vi "Pixie4SetUserPar.vi"(5 "Channel number":u16=2 max=3 step=1, 7 "Module number":u16 max=17 step=1, 10 "DownloadUserPar":bool, 11 "UploadUserPar":bool) -> (1 "trigger":bool, 2 "gain":dbl, 3 "Coincidence Pattern":u16=2048 format="%x")   [LabVIEW 2016]
uses:
  Drivers/Pixie4DLL.dll
panel:
  in  "?":bool
  in  "Module parameters":T1(tab)
  in  "Range":dbl=1.0 min=1.0 max=6.0 step=1.0
  out "Minimum coincidence\nwindow width [ns]":dbl=13.333333333333334 min=0.0
  in  "1 1 1 1":bool=TRUE
  in  "1 1 1 0":bool
  in  "1 1 0 1":bool
  in  "1 1 0 0":bool
  in  "1 0 1 1":bool=TRUE
  in  "1 0 1 0":bool
  in  "1 0 0 1":bool
  in  "1 0 0 0":bool
  in  "0 1 1 1":bool
  in  "0 1 1 0":bool
  in  "0 1 0 1":bool
  in  "0 1 0 0":bool
  in  "0 0 1 1":bool
  in  "0 0 1 0":bool
  in  "0 0 0 1":bool
  in  "0 0 0 0":bool
  in  "Actual coincidence\nwindow width [ns]":dbl=5000.0 min=0.0
  in  "CW options":dbl min=0.0 max=2.0 step=1.0
  in  "Module's local test adds to global test (local fail causes global fail)":bool
  in  "Accept event if global hit pattern passes global test (in PDM)":bool
  in  "Accept event if local pattern passes local test":bool=TRUE
  in  "PDM control pattern":i32 min=0 max=65535 step=1 format="%x"
  in  "Send local hit pattern to PDM in slot 2":bool
  in  "Module writes control pattern to PDM to immediate left":bool
  in  "Front panel contributes to STATUS line (wire-OR)":bool
  in  "Trigger share mode":i32 min=0 max=3 step=1
  in  "Front panel drives GFLT line (one module only)":bool
  in  "32 buffers per spill":bool=TRUE
  in  "Channel parameters":T2(tab)=enum."Analog signal conditioning"
  in  "Threshold":dbl=10.0 min=0.0
  in  "Flat top [µs]":dbl=0.08 min=0.0 max=0.8533 step=0.013333
  in  "Rise time [µs]":dbl=0.76 min=0.02666 max=0.8533 step=0.0133
  in  "Flat top [µs]":dbl=0.29333333333333333 min=0.0
  in  "Rise time [µs]":dbl=3.0933333333333337 min=0.0266 max=105.813
  in  "Integrator":dbl min=0.0 max=5.0 step=1.0
  in  "Inverted":bool
  in  "Estimate energy if not hit":bool
  in  "Latch local timestamp even in group trigger mode":bool
  in  "Threshold [%]":dbl=25.0 min=0.0 max=100.0 step=1.0
  in  "Compute constant fraction timing":bool
  in  "Histogram energies":bool=TRUE
  in  "GFLT required":bool
  in  "Trigger positive":bool=TRUE
  in  "Enable trigger":bool=TRUE
  in  "Read always":bool=TRUE
  in  "Good channel":bool=TRUE
  in  "Allow negative energy":bool
  in  "Respond to group triggers only":bool
  in  "Invert the GATE polarity to start the GATE Window":bool
  in  "Pause pileup inspection":bool
  in  "Invert pileup inspection":bool
  in  "Ignore out-of-range":bool
  in  "Disable pileup inspection":bool
  in  "Route VETO signal to be used for GATE":bool
  in  "Invert GATE polarity for acceptance":bool
  in  "GATE signal required to accept events":bool
  in  "PSA End [µs]":dbl min=0.0
  in  "PSA Start [µs]":dbl min=0.0
  in  "Delay [µs]":dbl min=0.0
  in  "Trace length [µs]":dbl min=0.0
  in  "Offset [V]":dbl=0.1180267333984375 min=0.0
  in  "Gain [V/V]":dbl=2.0 min=0.0
  in  "Tau [µs]":dbl=50.0 min=0.0
  in  "Binning factor":dbl=1.0 min=1.0 max=6.0 step=1.0
  in  "Minimum energy":dbl min=0.0
  in  "Gate Delay [µs]":dbl=0.013333333333333334 step=0.013333
  in  "Gate Window [µs]":dbl=0.013333333333333334 step=0.013333
  in  "Baseline Averaging":dbl=65534.0 min=0.0 max=65535.0 step=1.0
  in  "Baseline Cut":dbl=58.0 min=0.0 max=65535.0 step=1.0
  # "(Must also enable Upload button)"
  # "Energy Filter"
  # "Edit required hit patterns"
  # "Channels"
  # "Channels"
  # "3 2 1 0"
  # "3 2 1 0"
  # "0x"
  # "0: Increase for energy filter, never decrease\n1: Keep at required energy filter width\n2: Disregard energy filter requirement"
  # "0x"
  # "Trigger Filter"
  # "Energy Filter"
  # "Edit Channel Control Register A"
  # "Edit Channel Control Register C"
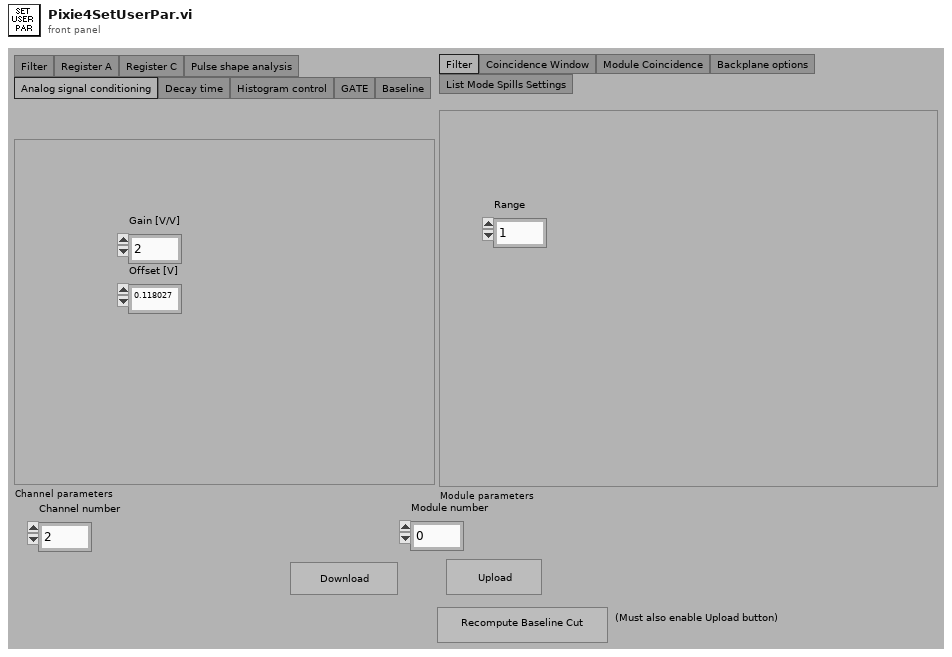
[diagram p1: front panel]
types:
  T1 = enum32{"Filter", "Coincidence Window", "Module Coincidence", "Backplane options", "List Mode Spills Settings"}
  T2 = enum32{"Filter", "Register A", "Register C", "Pulse shape analysis", "Analog signal conditioning", "Decay time", "Histogram control", "GATE", "Baseline"}
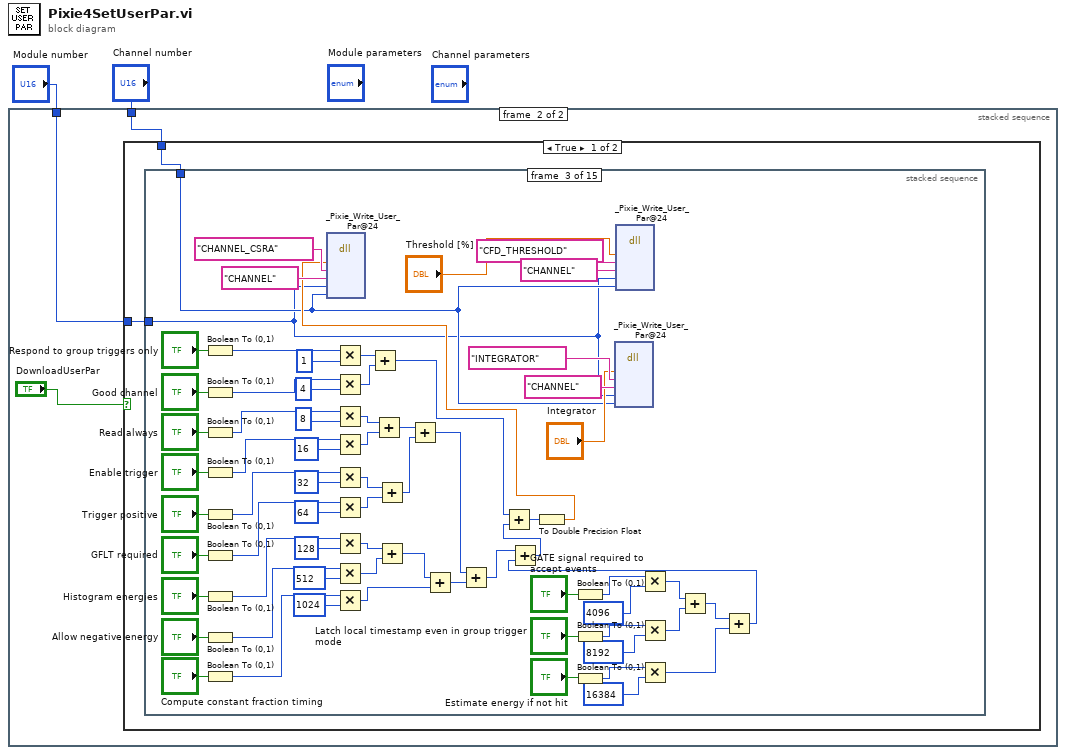
[diagram p0: block diagram]
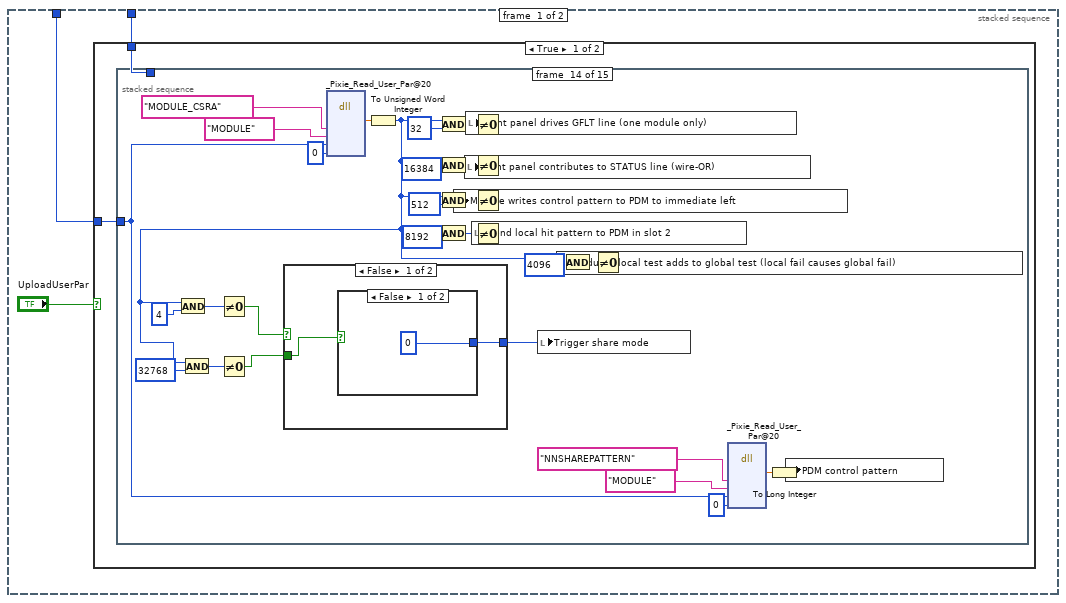
[diagram p2: hidden frame]
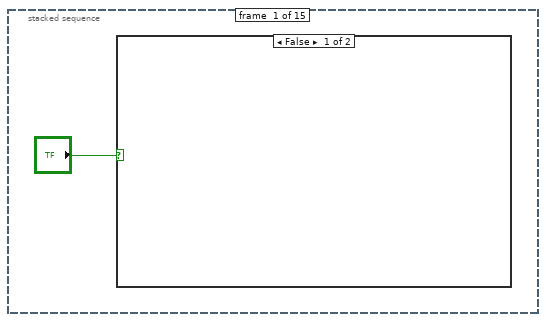
[diagram p3: hidden frame]
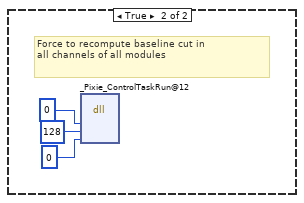
[diagram p4: hidden frame]
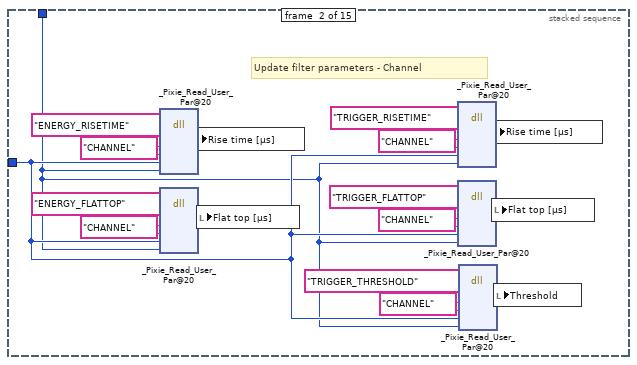
[diagram p5: hidden frame]
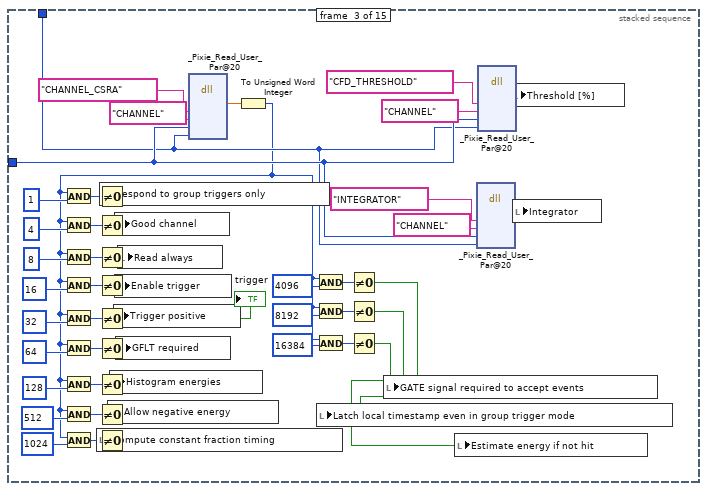
[diagram p6: hidden frame]
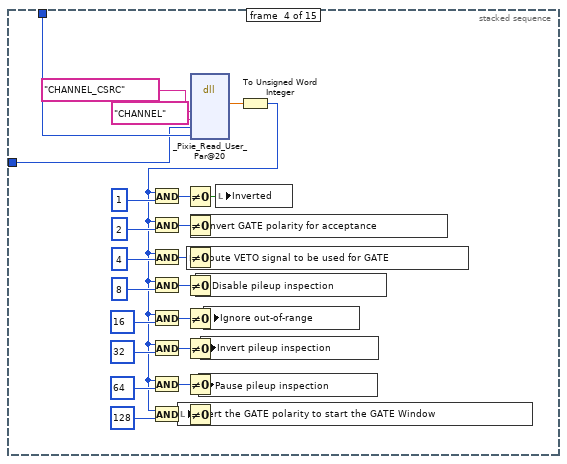
[diagram p7: hidden frame]
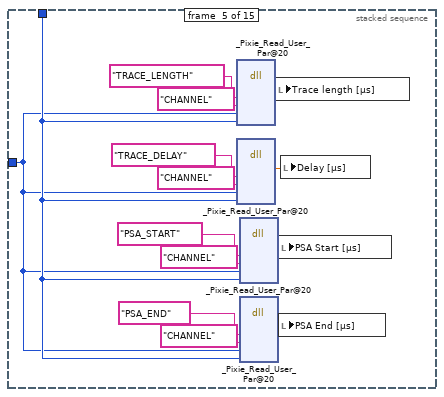
[diagram p8: hidden frame]
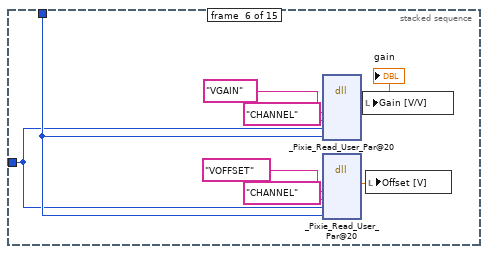
[diagram p9: hidden frame]
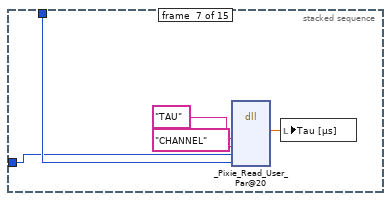
[diagram p10: hidden frame]
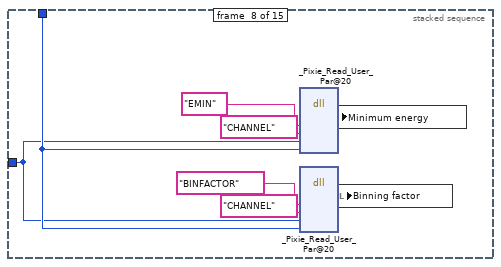
[diagram p11: hidden frame]
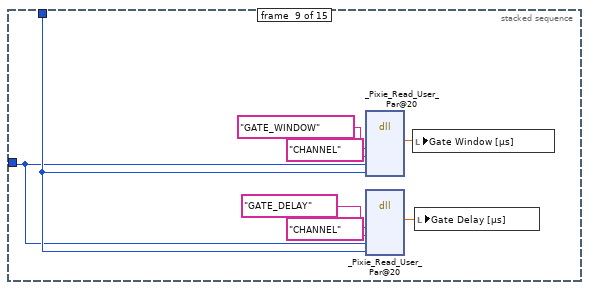
[diagram p12: hidden frame]
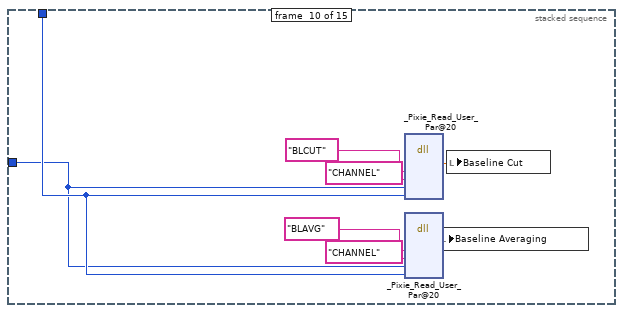
[diagram p13: hidden frame]
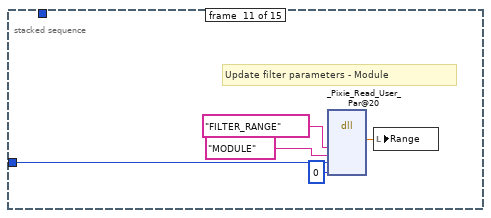
[diagram p14: hidden frame]
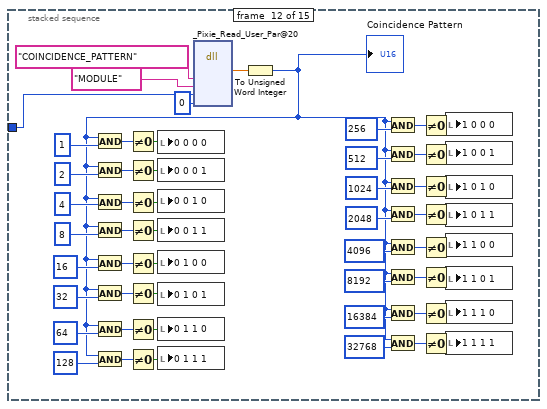
[diagram p15: hidden frame]
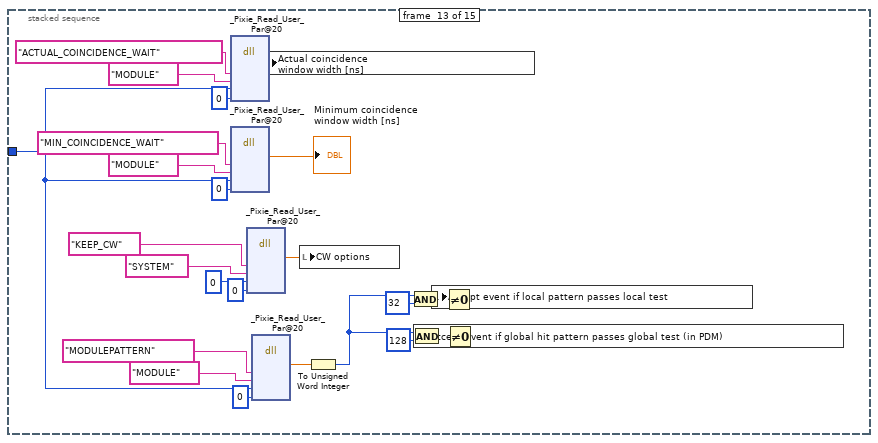
[diagram p16: hidden frame]
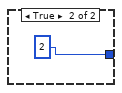
[diagram p17: hidden frame]
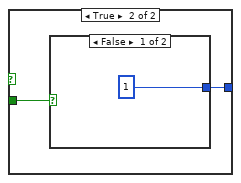
[diagram p18: hidden frame]
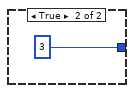
[diagram p19: hidden frame]
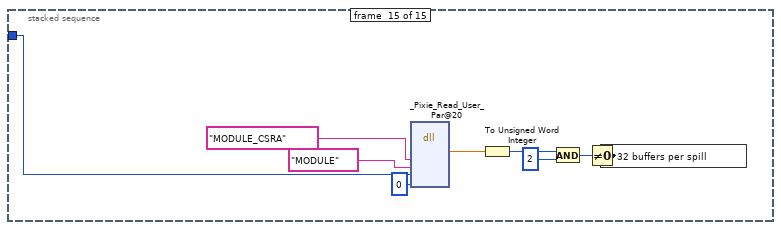
[diagram p20: hidden frame]
diagram:
  n1 = stacked-sequence {
    tunnel: "Module number" -> [w4 w294]
    tunnel: "Channel number" -> [w3 w293]
    frame #0 {
      n2 = case shown="True" "UploadUserPar" {
        tunnel: w4 -> [w7 _]
        tunnel: w3 -> [w6 _]
        frame True {
          n3 = stacked-sequence {
            tunnel: w7 -> [_ w14 w48 w86 w111 w123 w130 w136 w144 w156 w160 w213 w228 w254 w288]
            tunnel: w6 -> [_ w13 w47 w87 w112 w124 w131 w137 w145 w157 _ _ _ _ _]
            frame #0 {
              n4 = case shown="False" "?" {
                frame False {
                }
                frame True {
                  # "Force to recompute baseline cut in\nall channels of all modules"
                  n5 = dll-call lib="D:/Users/wymanm/Desktop/DAQuiri - 2017a/lois/Drivers/Pixie4DLL.dll" fn="_Pixie_ControlTaskRun@12"("ModNum"=0, "ControlTask"=128, "MaxPoll"=0) -> ()  [unwired: 7 in, 2 out]
                }
              }
            }
            frame #1 {
              # "Update filter parameters - Channel"
              n6 = dll-call lib="D:/Users/wymanm/Desktop/DAQuiri - 2017a/lois/Drivers/Pixie4DLL.dll" fn="_Pixie_Read_User_Par@20"("User_Par_Name"="ENERGY_RISETIME", "User_Par_Type"="CHANNEL", "ModNum"=w14, "ChanNum"=w13) -> ("User_Par_Value"=w26:dbl)  [unwired: 9 in, 2 out]
              n7 = dll-call lib="D:/Users/wymanm/Desktop/DAQuiri - 2017a/lois/Drivers/Pixie4DLL.dll" fn="_Pixie_Read_User_Par@20"("User_Par_Name"="ENERGY_FLATTOP", "User_Par_Type"="CHANNEL", "ModNum"=w14, "ChanNum"=w13) -> ("User_Par_Value"=w23:dbl)  [unwired: 9 in, 2 out]
              n8 = local write "Rise time [µs]"(w26) -> ()
              n9 = local write "Flat top [µs]"(w23) -> ()
              n10 = dll-call lib="D:/Users/wymanm/Desktop/DAQuiri - 2017a/lois/Drivers/Pixie4DLL.dll" fn="_Pixie_Read_User_Par@20"("User_Par_Name"="TRIGGER_RISETIME", "User_Par_Type"="CHANNEL", "ModNum"=w14, "ChanNum"=w13) -> ("User_Par_Value"=w18:dbl)  [unwired: 9 in, 2 out]
              n11 = dll-call lib="D:/Users/wymanm/Desktop/DAQuiri - 2017a/lois/Drivers/Pixie4DLL.dll" fn="_Pixie_Read_User_Par@20"("User_Par_Name"="TRIGGER_FLATTOP", "User_Par_Type"="CHANNEL", "ModNum"=w14, "ChanNum"=w13) -> ("User_Par_Value"=w17:dbl)  [unwired: 9 in, 2 out]
              n12 = dll-call lib="D:/Users/wymanm/Desktop/DAQuiri - 2017a/lois/Drivers/Pixie4DLL.dll" fn="_Pixie_Read_User_Par@20"("User_Par_Name"="TRIGGER_THRESHOLD", "User_Par_Type"="CHANNEL", "ModNum"=w14, "ChanNum"=w13) -> ("User_Par_Value"=w12:dbl)  [unwired: 9 in, 2 out]
              n13 = local write "Rise time [µs]"(w18) -> ()
              n14 = local write "Flat top [µs]"(w17) -> ()
              n15 = local write "Threshold"(w12) -> ()
            }
            frame #2 {
              n16 = dll-call lib="D:/Users/wymanm/Desktop/DAQuiri - 2017a/lois/Drivers/Pixie4DLL.dll" fn="_Pixie_Read_User_Par@20"("User_Par_Name"="CHANNEL_CSRA", "User_Par_Type"="CHANNEL", "ModNum"=w48, "ChanNum"=w47) -> ("User_Par_Value"=w68:dbl)  [unwired: 9 in, 2 out]
              n17 = To Unsigned Word Integer(number=w68) -> (unsigned 16bit integer=w32:u16)
              n18 = And(x=w32, y=1) -> (x .and. y?=w66:i32)
              n19 = And(x=w32, y=4) -> (x .and. y?=w63:i32)
              n20 = And(x=w32, y=8) -> (x .and. y?=w61:i32)
              n21 = And(x=w32, y=16) -> (x .and. y?=w59:i32)
              n22 = And(x=w32, y=32) -> (x .and. y?=w57:i32)
              n23 = And(x=w32, y=64) -> (x .and. y?=w55:i32)
              n24 = And(x=w32, y=128) -> (x .and. y?=w53:i32)
              n25 = And(x=w32, y=512) -> (x .and. y?=w51:i32)
              n26 = And(x=w32, y=1024) -> (x .and. y?=w49:i32)
              n27 = Not Equal To 0?(x=w66) -> (x != 0?=w65:bool)
              n28 = Not Equal To 0?(x=w63) -> (x != 0?=w46:bool)
              n29 = Not Equal To 0?(x=w61) -> (x != 0?=w45:bool)
              n30 = Not Equal To 0?(x=w59) -> (x != 0?=w44:bool)
              n31 = Not Equal To 0?(x=w57) -> (x != 0?=w43:bool)
              "trigger" <- w43
              n32 = Not Equal To 0?(x=w55) -> (x != 0?=w42:bool)
              n33 = Not Equal To 0?(x=w53) -> (x != 0?=w41:bool)
              n34 = Not Equal To 0?(x=w51) -> (x != 0?=w40:bool)
              n35 = Not Equal To 0?(x=w49) -> (x != 0?=w39:bool)
              n36 = local write "Compute constant fraction timing"(w39) -> ()
              n37 = local write "Respond to group triggers only"(w65) -> ()
              n38 = local write "Allow negative energy"(w40) -> ()
              n39 = local write "Histogram energies"(w41) -> ()
              n40 = local write "Trigger positive"(w43) -> ()
              n41 = local write "Good channel"(w46) -> ()
              n42 = local write "Enable trigger"(w44) -> ()
              n43 = local write "GFLT required"(w42) -> ()
              n44 = local write "Read always"(w45) -> ()
              n45 = And(x=w32, y=4096) -> (x .and. y?=w37:i32)
              n46 = And(x=w32, y=8192) -> (x .and. y?=w35:i32)
              n47 = And(x=w32, y=16384) -> (x .and. y?=w33:i32)
              n48 = Not Equal To 0?(x=w37) -> (x != 0?=w31:bool)
              n49 = Not Equal To 0?(x=w35) -> (x != 0?=w30:bool)
              n50 = local write "Latch local timestamp even in group trigger mode"(w30) -> ()
              n51 = Not Equal To 0?(x=w33) -> (x != 0?=w29:bool)
              n52 = local write "GATE signal required to accept events"(w31) -> ()
              n53 = local write "Estimate energy if not hit"(w29) -> ()
              n54 = dll-call lib="D:/Users/wymanm/Desktop/DAQuiri - 2017a/lois/Drivers/Pixie4DLL.dll" fn="_Pixie_Read_User_Par@20"("User_Par_Name"="INTEGRATOR", "User_Par_Type"="CHANNEL", "ModNum"=w48, "ChanNum"=w47) -> ("User_Par_Value"=w69:dbl)  [unwired: 9 in, 2 out]
              n55 = dll-call lib="D:/Users/wymanm/Desktop/DAQuiri - 2017a/lois/Drivers/Pixie4DLL.dll" fn="_Pixie_Read_User_Par@20"("User_Par_Name"="CFD_THRESHOLD", "User_Par_Type"="CHANNEL", "ModNum"=w48, "ChanNum"=w47) -> ("User_Par_Value"=w70:dbl)  [unwired: 9 in, 2 out]
              n56 = local write "Threshold [%]"(w70) -> ()
              n57 = local write "Integrator"(w69) -> ()
            }
            frame #3 {
              n58 = dll-call lib="D:/Users/wymanm/Desktop/DAQuiri - 2017a/lois/Drivers/Pixie4DLL.dll" fn="_Pixie_Read_User_Par@20"("User_Par_Name"="CHANNEL_CSRC", "User_Par_Type"="CHANNEL", "ModNum"=w86, "ChanNum"=w87) -> ("User_Par_Value"=w88:dbl)  [unwired: 9 in, 2 out]
              n59 = To Unsigned Word Integer(number=w88) -> (unsigned 16bit integer=w85:u16)
              n60 = And(x=w85, y=1) -> (x .and. y?=w105:i32)
              n61 = And(x=w85, y=2) -> (x .and. y?=w103:i32)
              n62 = And(x=w85, y=4) -> (x .and. y?=w101:i32)
              n63 = And(x=w85, y=8) -> (x .and. y?=w99:i32)
              n64 = And(x=w85, y=16) -> (x .and. y?=w97:i32)
              n65 = And(x=w85, y=32) -> (x .and. y?=w95:i32)
              n66 = And(x=w85, y=64) -> (x .and. y?=w93:i32)
              n67 = And(x=w85, y=128) -> (x .and. y?=w91:i32)
              n68 = Not Equal To 0?(x=w105) -> (x != 0?=w84:bool)
              n69 = Not Equal To 0?(x=w103) -> (x != 0?=w83:bool)
              n70 = Not Equal To 0?(x=w101) -> (x != 0?=w82:bool)
              n71 = Not Equal To 0?(x=w99) -> (x != 0?=w81:bool)
              n72 = Not Equal To 0?(x=w97) -> (x != 0?=w80:bool)
              n73 = Not Equal To 0?(x=w95) -> (x != 0?=w79:bool)
              n74 = Not Equal To 0?(x=w93) -> (x != 0?=w78:bool)
              n75 = Not Equal To 0?(x=w91) -> (x != 0?=w77:bool)
              n76 = local write "Invert the GATE polarity to start the GATE Window"(w77) -> ()
              n77 = local write "Route VETO signal to be used for GATE"(w82) -> ()
              n78 = local write "Invert GATE polarity for acceptance"(w83) -> ()
              n79 = local write "Disable pileup inspection"(w81) -> ()
              n80 = local write "Pause pileup inspection"(w78) -> ()
              n81 = local write "Invert pileup inspection"(w79) -> ()
              n82 = local write "Ignore out-of-range"(w80) -> ()
              n83 = local write "Inverted"(w84) -> ()
            }
            frame #4 {
              n84 = dll-call lib="D:/Users/wymanm/Desktop/DAQuiri - 2017a/lois/Drivers/Pixie4DLL.dll" fn="_Pixie_Read_User_Par@20"("User_Par_Name"="TRACE_LENGTH", "User_Par_Type"="CHANNEL", "ModNum"=w111, "ChanNum"=w112) -> ("User_Par_Value"=w110:dbl)  [unwired: 9 in, 2 out]
              n85 = dll-call lib="D:/Users/wymanm/Desktop/DAQuiri - 2017a/lois/Drivers/Pixie4DLL.dll" fn="_Pixie_Read_User_Par@20"("User_Par_Name"="TRACE_DELAY", "User_Par_Type"="CHANNEL", "ModNum"=w111, "ChanNum"=w112) -> ("User_Par_Value"=w109:dbl)  [unwired: 9 in, 2 out]
              n86 = dll-call lib="D:/Users/wymanm/Desktop/DAQuiri - 2017a/lois/Drivers/Pixie4DLL.dll" fn="_Pixie_Read_User_Par@20"("User_Par_Name"="PSA_START", "User_Par_Type"="CHANNEL", "ModNum"=w111, "ChanNum"=w112) -> ("User_Par_Value"=w108:dbl)  [unwired: 9 in, 2 out]
              n87 = dll-call lib="D:/Users/wymanm/Desktop/DAQuiri - 2017a/lois/Drivers/Pixie4DLL.dll" fn="_Pixie_Read_User_Par@20"("User_Par_Name"="PSA_END", "User_Par_Type"="CHANNEL", "ModNum"=w111, "ChanNum"=w112) -> ("User_Par_Value"=w107:dbl)  [unwired: 9 in, 2 out]
              n88 = local write "Trace length [µs]"(w110) -> ()
              n89 = local write "PSA Start [µs]"(w108) -> ()
              n90 = local write "PSA End [µs]"(w107) -> ()
              n91 = local write "Delay [µs]"(w109) -> ()
            }
            frame #5 {
              n92 = dll-call lib="D:/Users/wymanm/Desktop/DAQuiri - 2017a/lois/Drivers/Pixie4DLL.dll" fn="_Pixie_Read_User_Par@20"("User_Par_Name"="VGAIN", "User_Par_Type"="CHANNEL", "ModNum"=w123, "ChanNum"=w124) -> ("User_Par_Value"=w122:dbl)  [unwired: 9 in, 2 out]
              "gain" <- w122
              n93 = dll-call lib="D:/Users/wymanm/Desktop/DAQuiri - 2017a/lois/Drivers/Pixie4DLL.dll" fn="_Pixie_Read_User_Par@20"("User_Par_Name"="VOFFSET", "User_Par_Type"="CHANNEL", "ModNum"=w123, "ChanNum"=w124) -> ("User_Par_Value"=w121:dbl)  [unwired: 9 in, 2 out]
              n94 = local write "Gain [V/V]"(w122) -> ()
              n95 = local write "Offset [V]"(w121) -> ()
            }
            frame #6 {
              n96 = dll-call lib="D:/Users/wymanm/Desktop/DAQuiri - 2017a/lois/Drivers/Pixie4DLL.dll" fn="_Pixie_Read_User_Par@20"("User_Par_Name"="TAU", "User_Par_Type"="CHANNEL", "ModNum"=w130, "ChanNum"=w131) -> ("User_Par_Value"=w129:dbl)  [unwired: 9 in, 2 out]
              n97 = local write "Tau [µs]"(w129) -> ()
            }
            frame #7 {
              n98 = dll-call lib="D:/Users/wymanm/Desktop/DAQuiri - 2017a/lois/Drivers/Pixie4DLL.dll" fn="_Pixie_Read_User_Par@20"("User_Par_Name"="EMIN", "User_Par_Type"="CHANNEL", "ModNum"=w136, "ChanNum"=w137) -> ("User_Par_Value"=w135:dbl)  [unwired: 9 in, 2 out]
              n99 = dll-call lib="D:/Users/wymanm/Desktop/DAQuiri - 2017a/lois/Drivers/Pixie4DLL.dll" fn="_Pixie_Read_User_Par@20"("User_Par_Name"="BINFACTOR", "User_Par_Type"="CHANNEL", "ModNum"=w136, "ChanNum"=w137) -> ("User_Par_Value"=w134:dbl)  [unwired: 9 in, 2 out]
              n100 = local write "Minimum energy"(w135) -> ()
              n101 = local write "Binning factor"(w134) -> ()
            }
            frame #8 {
              n102 = dll-call lib="D:/Users/wymanm/Desktop/DAQuiri - 2017a/lois/Drivers/Pixie4DLL.dll" fn="_Pixie_Read_User_Par@20"("User_Par_Name"="GATE_WINDOW", "User_Par_Type"="CHANNEL", "ModNum"=w144, "ChanNum"=w145) -> ("User_Par_Value"=w143:dbl)  [unwired: 9 in, 2 out]
              n103 = dll-call lib="D:/Users/wymanm/Desktop/DAQuiri - 2017a/lois/Drivers/Pixie4DLL.dll" fn="_Pixie_Read_User_Par@20"("User_Par_Name"="GATE_DELAY", "User_Par_Type"="CHANNEL", "ModNum"=w144, "ChanNum"=w145) -> ("User_Par_Value"=w142:dbl)  [unwired: 9 in, 2 out]
              n104 = local write "Gate Window [µs]"(w143) -> ()
              n105 = local write "Gate Delay [µs]"(w142) -> ()
            }
            frame #9 {
              n106 = dll-call lib="D:/Users/wymanm/Desktop/DAQuiri - 2017a/lois/Drivers/Pixie4DLL.dll" fn="_Pixie_Read_User_Par@20"("User_Par_Name"="BLCUT", "User_Par_Type"="CHANNEL", "ModNum"=w156, "ChanNum"=w157) -> ("User_Par_Value"=w151:dbl)  [unwired: 9 in, 2 out]
              n107 = dll-call lib="D:/Users/wymanm/Desktop/DAQuiri - 2017a/lois/Drivers/Pixie4DLL.dll" fn="_Pixie_Read_User_Par@20"("User_Par_Name"="BLAVG", "User_Par_Type"="CHANNEL", "ModNum"=w156, "ChanNum"=w157) -> ("User_Par_Value"=w150:dbl)  [unwired: 9 in, 2 out]
              n108 = local write "Baseline Averaging"(w150) -> ()
              n109 = local write "Baseline Cut"(w151) -> ()
            }
            frame #10 {
              # "Update filter parameters - Module"
              n110 = dll-call lib="D:/Users/wymanm/Desktop/DAQuiri - 2017a/lois/Drivers/Pixie4DLL.dll" fn="_Pixie_Read_User_Par@20"("User_Par_Name"="FILTER_RANGE", "User_Par_Type"="MODULE", "ModNum"=w160, "ChanNum"=0) -> ("User_Par_Value"=w158:dbl)  [unwired: 9 in, 2 out]
              n111 = local write "Range"(w158) -> ()
            }
            frame #11 {
              n112 = dll-call lib="D:/Users/wymanm/Desktop/DAQuiri - 2017a/lois/Drivers/Pixie4DLL.dll" fn="_Pixie_Read_User_Par@20"("User_Par_Name"="COINCIDENCE_PATTERN", "User_Par_Type"="MODULE", "ModNum"=w213, "ChanNum"=0) -> ("User_Par_Value"=w180:dbl)  [unwired: 9 in, 2 out]
              n113 = To Unsigned Word Integer(number=w180) -> (unsigned 16bit integer=w163:u16)
              "Coincidence Pattern" <- w163
              n114 = And(x=w163, y=1) -> (x .and. y?=w211:i32)
              n115 = And(x=w163, y=2) -> (x .and. y?=w209:i32)
              n116 = And(x=w163, y=4) -> (x .and. y?=w207:i32)
              n117 = And(x=w163, y=8) -> (x .and. y?=w205:i32)
              n118 = And(x=w163, y=16) -> (x .and. y?=w203:i32)
              n119 = And(x=w163, y=32) -> (x .and. y?=w201:i32)
              n120 = And(x=w163, y=64) -> (x .and. y?=w199:i32)
              n121 = And(x=w163, y=128) -> (x .and. y?=w197:i32)
              n122 = Not Equal To 0?(x=w211) -> (x != 0?=w179:bool)
              n123 = Not Equal To 0?(x=w209) -> (x != 0?=w178:bool)
              n124 = Not Equal To 0?(x=w207) -> (x != 0?=w177:bool)
              n125 = Not Equal To 0?(x=w205) -> (x != 0?=w176:bool)
              n126 = Not Equal To 0?(x=w203) -> (x != 0?=w175:bool)
              n127 = Not Equal To 0?(x=w201) -> (x != 0?=w174:bool)
              n128 = Not Equal To 0?(x=w199) -> (x != 0?=w173:bool)
              n129 = Not Equal To 0?(x=w197) -> (x != 0?=w172:bool)
              n130 = local write "0 0 0 0"(w179) -> ()
              n131 = local write "0 0 0 1"(w178) -> ()
              n132 = local write "0 0 1 0"(w177) -> ()
              n133 = local write "0 0 1 1"(w176) -> ()
              n134 = local write "0 1 0 0"(w175) -> ()
              n135 = local write "0 1 0 1"(w174) -> ()
              n136 = local write "0 1 1 0"(w173) -> ()
              n137 = local write "0 1 1 1"(w172) -> ()
              n138 = And(x=w163, y=256) -> (x .and. y?=w195:i32)
              n139 = And(x=w163, y=512) -> (x .and. y?=w193:i32)
              n140 = And(x=w163, y=1024) -> (x .and. y?=w191:i32)
              n141 = And(x=w163, y=2048) -> (x .and. y?=w189:i32)
              n142 = And(x=w163, y=4096) -> (x .and. y?=w187:i32)
              n143 = And(x=w163, y=8192) -> (x .and. y?=w185:i32)
              n144 = And(x=w163, y=16384) -> (x .and. y?=w183:i32)
              n145 = And(x=w163, y=32768) -> (x .and. y?=w181:i32)
              n146 = Not Equal To 0?(x=w195) -> (x != 0?=w171:bool)
              n147 = Not Equal To 0?(x=w193) -> (x != 0?=w170:bool)
              n148 = Not Equal To 0?(x=w191) -> (x != 0?=w169:bool)
              n149 = Not Equal To 0?(x=w189) -> (x != 0?=w168:bool)
              n150 = Not Equal To 0?(x=w187) -> (x != 0?=w167:bool)
              n151 = Not Equal To 0?(x=w185) -> (x != 0?=w166:bool)
              n152 = Not Equal To 0?(x=w183) -> (x != 0?=w165:bool)
              n153 = Not Equal To 0?(x=w181) -> (x != 0?=w164:bool)
              n154 = local write "1 0 0 0"(w171) -> ()
              n155 = local write "1 0 0 1"(w170) -> ()
              n156 = local write "1 0 1 0"(w169) -> ()
              n157 = local write "1 0 1 1"(w168) -> ()
              n158 = local write "1 1 0 0"(w167) -> ()
              n159 = local write "1 1 0 1"(w166) -> ()
              n160 = local write "1 1 1 0"(w165) -> ()
              n161 = local write "1 1 1 1"(w164) -> ()
            }
            frame #12 {
              n162 = dll-call lib="D:/Users/wymanm/Desktop/DAQuiri - 2017a/lois/Drivers/Pixie4DLL.dll" fn="_Pixie_Read_User_Par@20"("User_Par_Name"="ACTUAL_COINCIDENCE_WAIT", "User_Par_Type"="MODULE", "ModNum"=w228, "ChanNum"=0) -> ("User_Par_Value"=w218:dbl)  [unwired: 9 in, 2 out]
              n163 = dll-call lib="D:/Users/wymanm/Desktop/DAQuiri - 2017a/lois/Drivers/Pixie4DLL.dll" fn="_Pixie_Read_User_Par@20"("User_Par_Name"="MIN_COINCIDENCE_WAIT", "User_Par_Type"="MODULE", "ModNum"=w228, "ChanNum"=0) -> ("User_Par_Value"=→"Minimum coincidence\nwindow width [ns]":dbl)  [unwired: 9 in, 2 out]
              n164 = dll-call lib="D:/Users/wymanm/Desktop/DAQuiri - 2017a/lois/Drivers/Pixie4DLL.dll" fn="_Pixie_Read_User_Par@20"("User_Par_Name"="KEEP_CW", "User_Par_Type"="SYSTEM", "ModNum"=0, "ChanNum"=0) -> ("User_Par_Value"=w217:dbl)  [unwired: 9 in, 2 out]
              n165 = dll-call lib="D:/Users/wymanm/Desktop/DAQuiri - 2017a/lois/Drivers/Pixie4DLL.dll" fn="_Pixie_Read_User_Par@20"("User_Par_Name"="MODULEPATTERN", "User_Par_Type"="MODULE", "ModNum"=w228, "ChanNum"=0) -> ("User_Par_Value"=w225:dbl)  [unwired: 9 in, 2 out]
              n166 = local write "Actual coincidence\nwindow width [ns]"(w218) -> ()
              n167 = local write "CW options"(w217) -> ()
              n168 = To Unsigned Word Integer(number=w225) -> (unsigned 16bit integer=w221:u16)
              n169 = And(x=w221, y=32) -> (x .and. y?=w226:i32)
              n170 = And(x=w221, y=128) -> (x .and. y?=w223:i32)
              n171 = Not Equal To 0?(x=w226) -> (x != 0?=w219:bool)
              n172 = local write "Accept event if local pattern passes local test"(w219) -> ()
              n173 = Not Equal To 0?(x=w223) -> (x != 0?=w222:bool)
              n174 = local write "Accept event if global hit pattern passes global test (in PDM)"(w222) -> ()
            }
            frame #13 {
              n175 = dll-call lib="D:/Users/wymanm/Desktop/DAQuiri - 2017a/lois/Drivers/Pixie4DLL.dll" fn="_Pixie_Read_User_Par@20"("User_Par_Name"="MODULE_CSRA", "User_Par_Type"="MODULE", "ModNum"=w254, "ChanNum"=0) -> ("User_Par_Value"=w269:dbl)  [unwired: 9 in, 2 out]
              n176 = To Unsigned Word Integer(number=w269) -> (unsigned 16bit integer=w243:u16)
              n177 = And(x=w243, y=4) -> (x .and. y?=w250:i32)
              n178 = And(x=w243, y=32768) -> (x .and. y?=w249:i32)
              n179 = Not Equal To 0?(x=w250) -> (x != 0?=w248:bool)
              n180 = Not Equal To 0?(x=w249) -> (x != 0?=w247:bool)
              n181 = case shown="False" w248 {
                tunnel: w247 -> [w276 w280]
                tunnel: [w275 w279] -> w246
                frame False {
                  n182 = case shown="False" w276 {
                    tunnel: [0 2] -> w275
                    frame False {
                    }
                    frame True {
                    }
                  }
                }
                frame True {
                  n183 = case shown="False" w280 {
                    tunnel: [1 3] -> w279
                    frame False {
                    }
                    frame True {
                    }
                  }
                }
              }
              n184 = And(x=w243, y=32) -> (x .and. y?=w270:i32)
              n185 = And(x=w243, y=16384) -> (x .and. y?=w267:i32)
              n186 = And(x=w243, y=512) -> (x .and. y?=w265:i32)
              n187 = And(x=w243, y=8192) -> (x .and. y?=w263:i32)
              n188 = Not Equal To 0?(x=w270) -> (x != 0?=w261:bool)
              n189 = local write "Front panel drives GFLT line (one module only)"(w261) -> ()
              n190 = Not Equal To 0?(x=w267) -> (x != 0?=w262:bool)
              n191 = local write "Front panel contributes to STATUS line (wire-OR)"(w262) -> ()
              n192 = Not Equal To 0?(x=w265) -> (x != 0?=w260:bool)
              n193 = local write "Module writes control pattern to PDM to immediate left"(w260) -> ()
              n194 = Not Equal To 0?(x=w263) -> (x != 0?=w259:bool)
              n195 = local write "Send local hit pattern to PDM in slot 2"(w259) -> ()
              n196 = local write "Trigger share mode"(w246) -> ()
              n197 = And(x=w243, y=4096) -> (x .and. y?=w244:i32)
              n198 = Not Equal To 0?(x=w244) -> (x != 0?=w242:bool)
              n199 = local write "Module's local test adds to global test (local fail causes global fail)"(w242) -> ()
              n200 = dll-call lib="D:/Users/wymanm/Desktop/DAQuiri - 2017a/lois/Drivers/Pixie4DLL.dll" fn="_Pixie_Read_User_Par@20"("User_Par_Name"="NNSHAREPATTERN", "User_Par_Type"="MODULE", "ModNum"=w254, "ChanNum"=0) -> ("User_Par_Value"=w255:dbl)  [unwired: 9 in, 2 out]
              n201 = To Long Integer(number=w255) -> (32bit integer=w253:i32)
              n202 = local write "PDM control pattern"(w253) -> ()
            }
            frame #14 {
              n203 = dll-call lib="D:/Users/wymanm/Desktop/DAQuiri - 2017a/lois/Drivers/Pixie4DLL.dll" fn="_Pixie_Read_User_Par@20"("User_Par_Name"="MODULE_CSRA", "User_Par_Type"="MODULE", "ModNum"=w288, "ChanNum"=0) -> ("User_Par_Value"=w284:dbl)  [unwired: 9 in, 2 out]
              n204 = To Unsigned Word Integer(number=w284) -> (unsigned 16bit integer=w285:u16)
              n205 = And(x=w285, y=2) -> (x .and. y?=w286:i32)
              n206 = Not Equal To 0?(x=w286) -> (x != 0?=w283:bool)
              n207 = local write "32 buffers per spill"(w283) -> ()
            }
          }
        }
        frame False {
        }
      }
    }
    frame #1 {
      n208 = case shown="True" "DownloadUserPar" {
        tunnel: w294 -> [w296 _]
        tunnel: w293 -> [w295 _]
        frame True {
          n209 = stacked-sequence {
            tunnel: w296 -> [w297 w314 w350 w396 w443 w455 w462 w468 w476 w484 w492 w575 w579 w638 w677]
            tunnel: w295 -> [_ w313 w351 w395 w444 w456 w463 w469 w475 w485 _ _ _ _ _]
            frame #0 {
              n210 = stacked-sequence {
                tunnel: w297 -> [_ w303]
                frame #0 {
                  n211 = dll-call lib="D:/Users/wymanm/Desktop/DAQuiri - 2017a/lois/Drivers/Pixie4DLL.dll" fn="_Pixie_Write_User_Par@24"("User_Par_Value"="CW options", "User_Par_Name"="KEEP_CW", "User_Par_Type"="SYSTEM", "ModNum"=0, "ChanNum"=0) -> ()  [unwired: 9 in, 2 out]
                }
                frame #1 {
                  n212 = dll-call lib="D:/Users/wymanm/Desktop/DAQuiri - 2017a/lois/Drivers/Pixie4DLL.dll" fn="_Pixie_Write_User_Par@24"("User_Par_Value"="Actual coincidence\nwindow width [ns]", "User_Par_Name"="ACTUAL_COINCIDENCE_WAIT", "User_Par_Type"="MODULE", "ModNum"=w303, "ChanNum"=0) -> ()  [unwired: 9 in, 2 out]
                }
              }
            }
            frame #1 {
              # "Download filter parameters - Channel"
              n213 = dll-call lib="D:/Users/wymanm/Desktop/DAQuiri - 2017a/lois/Drivers/Pixie4DLL.dll" fn="_Pixie_Write_User_Par@24"("User_Par_Value"="Rise time [µs]", "User_Par_Name"="ENERGY_RISETIME", "User_Par_Type"="CHANNEL", "ModNum"=w314, "ChanNum"=w313) -> ()  [unwired: 9 in, 2 out]
              n214 = dll-call lib="D:/Users/wymanm/Desktop/DAQuiri - 2017a/lois/Drivers/Pixie4DLL.dll" fn="_Pixie_Write_User_Par@24"("User_Par_Value"="Flat top [µs]", "User_Par_Name"="ENERGY_FLATTOP", "User_Par_Type"="CHANNEL", "ModNum"=w314, "ChanNum"=w313) -> ()  [unwired: 9 in, 2 out]
              n215 = dll-call lib="D:/Users/wymanm/Desktop/DAQuiri - 2017a/lois/Drivers/Pixie4DLL.dll" fn="_Pixie_Write_User_Par@24"("User_Par_Value"="Rise time [µs]", "User_Par_Name"="TRIGGER_RISETIME", "User_Par_Type"="CHANNEL", "ModNum"=w314, "ChanNum"=w313) -> ()  [unwired: 9 in, 2 out]
              n216 = dll-call lib="D:/Users/wymanm/Desktop/DAQuiri - 2017a/lois/Drivers/Pixie4DLL.dll" fn="_Pixie_Write_User_Par@24"("User_Par_Value"="Flat top [µs]", "User_Par_Name"="TRIGGER_FLATTOP", "User_Par_Type"="CHANNEL", "ModNum"=w314, "ChanNum"=w313) -> ()  [unwired: 9 in, 2 out]
              n217 = dll-call lib="D:/Users/wymanm/Desktop/DAQuiri - 2017a/lois/Drivers/Pixie4DLL.dll" fn="_Pixie_Write_User_Par@24"("User_Par_Value"="Threshold", "User_Par_Name"="TRIGGER_THRESHOLD", "User_Par_Type"="CHANNEL", "ModNum"=w314, "ChanNum"=w313) -> ()  [unwired: 9 in, 2 out]
            }
            frame #2 {
              n218 = Boolean To (0,1)(Boolean="Respond to group triggers only") -> (0, 1=w377:i16)
              n219 = Boolean To (0,1)(Boolean="Good channel") -> (0, 1=w376:i16)
              n220 = Boolean To (0,1)(Boolean="Read always") -> (0, 1=w375:i16)
              n221 = Boolean To (0,1)(Boolean="Enable trigger") -> (0, 1=w374:i16)
              n222 = Boolean To (0,1)(Boolean="Trigger positive") -> (0, 1=w373:i16)
              n223 = Boolean To (0,1)(Boolean="GFLT required") -> (0, 1=w372:i16)
              n224 = Boolean To (0,1)(Boolean="Histogram energies") -> (0, 1=w371:i16)
              n225 = Boolean To (0,1)(Boolean="Allow negative energy") -> (0, 1=w370:i16)
              n226 = Boolean To (0,1)(Boolean="Compute constant fraction timing") -> (0, 1=w369:i16)
              n227 = Multiply(x=w377, y=1) -> (x*y=w368:i32)
              n228 = Multiply(x=w376, y=4) -> (x*y=w367:i32)
              n229 = Multiply(x=w375, y=8) -> (x*y=w366:i32)
              n230 = Multiply(x=w374, y=16) -> (x*y=w365:i32)
              n231 = Multiply(x=w373, y=32) -> (x*y=w364:i32)
              n232 = Multiply(x=w372, y=64) -> (x*y=w363:i32)
              n233 = Multiply(x=w371, y=128) -> (x*y=w362:i32)
              n234 = Multiply(x=w370, y=512) -> (x*y=w361:i32)
              n235 = Multiply(x=w369, y=1024) -> (x*y=w359:i32)
              n236 = Add(x=w368, y=w367) -> (x+y=w352:i32)
              n237 = Add(x=w366, y=w365) -> (x+y=w358:i32)
              n238 = Add(x=w364, y=w363) -> (x+y=w357:i32)
              n239 = Add(x=w362, y=w361) -> (x+y=w360:i32)
              n240 = Add(x=w358, y=w357) -> (x+y=w355:i32)
              n241 = Add(x=w360, y=w359) -> (x+y=w356:i32)
              n242 = Add(x=w355, y=w356) -> (x+y=w328:i32)
              n243 = Boolean To (0,1)(Boolean="GATE signal required to accept events") -> (0, 1=w338:i16)
              n244 = Boolean To (0,1)(Boolean="Latch local timestamp even in group trigger mode") -> (0, 1=w337:i16)
              n245 = Boolean To (0,1)(Boolean="Estimate energy if not hit") -> (0, 1=w336:i16)
              n246 = dll-call lib="D:/Users/wymanm/Desktop/DAQuiri - 2017a/lois/Drivers/Pixie4DLL.dll" fn="_Pixie_Write_User_Par@24"("User_Par_Value"="Integrator", "User_Par_Name"="INTEGRATOR", "User_Par_Type"="CHANNEL", "ModNum"=w350, "ChanNum"=w351) -> ()  [unwired: 9 in, 2 out]
              n247 = dll-call lib="D:/Users/wymanm/Desktop/DAQuiri - 2017a/lois/Drivers/Pixie4DLL.dll" fn="_Pixie_Write_User_Par@24"("User_Par_Value"="Threshold [%]", "User_Par_Name"="CFD_THRESHOLD", "User_Par_Type"="CHANNEL", "ModNum"=w350, "ChanNum"=w351) -> ()  [unwired: 9 in, 2 out]
              n248 = Multiply(x=w338, y=4096) -> (x*y=w332:i32)
              n249 = Multiply(x=w337, y=8192) -> (x*y=w331:i32)
              n250 = Multiply(x=w336, y=16384) -> (x*y=w329:i32)
              n251 = Add(x=w332, y=w331) -> (x+y=w330:i32)
              n252 = Add(x=w330, y=w329) -> (x+y=w327:i32)
              n253 = Add(x=w328, y=w327) -> (x+y=w326:i32)
              n254 = Add(x=w352, y=w326) -> (x+y=w354:i32)
              n255 = To Double Precision Float(number=w354) -> (double precision float=w353:dbl)
              n256 = dll-call lib="D:/Users/wymanm/Desktop/DAQuiri - 2017a/lois/Drivers/Pixie4DLL.dll" fn="_Pixie_Write_User_Par@24"("User_Par_Value"=w353, "User_Par_Name"="CHANNEL_CSRA", "User_Par_Type"="CHANNEL", "ModNum"=w350, "ChanNum"=w351) -> ()  [unwired: 9 in, 2 out]
            }
            frame #3 {
              n257 = Boolean To (0,1)(Boolean="Inverted") -> (0, 1=w430:i16)
              n258 = Boolean To (0,1)(Boolean="Invert GATE polarity for acceptance") -> (0, 1=w429:i16)
              n259 = Boolean To (0,1)(Boolean="Route VETO signal to be used for GATE") -> (0, 1=w428:i16)
              n260 = Boolean To (0,1)(Boolean="Disable pileup inspection") -> (0, 1=w427:i16)
              n261 = Boolean To (0,1)(Boolean="Ignore out-of-range") -> (0, 1=w426:i16)
              n262 = Boolean To (0,1)(Boolean="Invert pileup inspection") -> (0, 1=w425:i16)
              n263 = Boolean To (0,1)(Boolean="Pause pileup inspection") -> (0, 1=w424:i16)
              n264 = Boolean To (0,1)(Boolean="Invert the GATE polarity to start the GATE Window") -> (0, 1=w423:i16)
              n265 = Multiply(x=w430, y=1) -> (x*y=w422:i32)
              n266 = Multiply(x=w429, y=2) -> (x*y=w421:i32)
              n267 = Multiply(x=w428, y=4) -> (x*y=w420:i32)
              n268 = Multiply(x=w427, y=8) -> (x*y=w419:i32)
              n269 = Multiply(x=w426, y=16) -> (x*y=w418:i32)
              n270 = Multiply(x=w425, y=32) -> (x*y=w417:i32)
              n271 = Multiply(x=w424, y=64) -> (x*y=w416:i32)
              n272 = Multiply(x=w423, y=128) -> (x*y=w415:i32)
              n273 = Add(x=w422, y=w421) -> (x+y=w402:i32)
              n274 = Add(x=w420, y=w419) -> (x+y=w414:i32)
              n275 = Add(x=w418, y=w417) -> (x+y=w413:i32)
              n276 = Add(x=w416, y=w415) -> (x+y=w403:i32)
              n277 = Add(x=w414, y=w413) -> (x+y=w412:i32)
              n278 = Add(x=w412, y=w403) -> (x+y=w401:i32)
              n279 = Add(x=w402, y=w401) -> (x+y=w398:i32)
              n280 = To Double Precision Float(number=w398) -> (double precision float=w397:dbl)
              n281 = dll-call lib="D:/Users/wymanm/Desktop/DAQuiri - 2017a/lois/Drivers/Pixie4DLL.dll" fn="_Pixie_Write_User_Par@24"("User_Par_Value"=w397, "User_Par_Name"="CHANNEL_CSRC", "User_Par_Type"="CHANNEL", "ModNum"=w396, "ChanNum"=w395) -> ()  [unwired: 9 in, 2 out]
            }
            frame #4 {
              n282 = dll-call lib="D:/Users/wymanm/Desktop/DAQuiri - 2017a/lois/Drivers/Pixie4DLL.dll" fn="_Pixie_Write_User_Par@24"("User_Par_Value"="Trace length [µs]", "User_Par_Name"="TRACE_LENGTH", "User_Par_Type"="CHANNEL", "ModNum"=w443, "ChanNum"=w444) -> ()  [unwired: 9 in, 2 out]
              n283 = dll-call lib="D:/Users/wymanm/Desktop/DAQuiri - 2017a/lois/Drivers/Pixie4DLL.dll" fn="_Pixie_Write_User_Par@24"("User_Par_Value"="Delay [µs]", "User_Par_Name"="TRACE_DELAY", "User_Par_Type"="CHANNEL", "ModNum"=w443, "ChanNum"=w444) -> ()  [unwired: 9 in, 2 out]
              n284 = dll-call lib="D:/Users/wymanm/Desktop/DAQuiri - 2017a/lois/Drivers/Pixie4DLL.dll" fn="_Pixie_Write_User_Par@24"("User_Par_Value"="PSA Start [µs]", "User_Par_Name"="PSA_START", "User_Par_Type"="CHANNEL", "ModNum"=w443, "ChanNum"=w444) -> ()  [unwired: 9 in, 2 out]
              n285 = dll-call lib="D:/Users/wymanm/Desktop/DAQuiri - 2017a/lois/Drivers/Pixie4DLL.dll" fn="_Pixie_Write_User_Par@24"("User_Par_Value"="PSA End [µs]", "User_Par_Name"="PSA_END", "User_Par_Type"="CHANNEL", "ModNum"=w443, "ChanNum"=w444) -> ()  [unwired: 9 in, 2 out]
            }
            frame #5 {
              n286 = dll-call lib="D:/Users/wymanm/Desktop/DAQuiri - 2017a/lois/Drivers/Pixie4DLL.dll" fn="_Pixie_Write_User_Par@24"("User_Par_Value"="Gain [V/V]", "User_Par_Name"="VGAIN", "User_Par_Type"="CHANNEL", "ModNum"=w455, "ChanNum"=w456) -> ()  [unwired: 9 in, 2 out]
              n287 = dll-call lib="D:/Users/wymanm/Desktop/DAQuiri - 2017a/lois/Drivers/Pixie4DLL.dll" fn="_Pixie_Write_User_Par@24"("User_Par_Value"="Offset [V]", "User_Par_Name"="VOFFSET", "User_Par_Type"="CHANNEL", "ModNum"=w455, "ChanNum"=w456) -> ()  [unwired: 9 in, 2 out]
            }
            frame #6 {
              n288 = dll-call lib="D:/Users/wymanm/Desktop/DAQuiri - 2017a/lois/Drivers/Pixie4DLL.dll" fn="_Pixie_Write_User_Par@24"("User_Par_Value"="Tau [µs]", "User_Par_Name"="TAU", "User_Par_Type"="CHANNEL", "ModNum"=w462, "ChanNum"=w463) -> ()  [unwired: 9 in, 2 out]
            }
            frame #7 {
              n289 = dll-call lib="D:/Users/wymanm/Desktop/DAQuiri - 2017a/lois/Drivers/Pixie4DLL.dll" fn="_Pixie_Write_User_Par@24"("User_Par_Value"="Minimum energy", "User_Par_Name"="EMIN", "User_Par_Type"="CHANNEL", "ModNum"=w468, "ChanNum"=w469) -> ()  [unwired: 9 in, 2 out]
              n290 = dll-call lib="D:/Users/wymanm/Desktop/DAQuiri - 2017a/lois/Drivers/Pixie4DLL.dll" fn="_Pixie_Write_User_Par@24"("User_Par_Value"="Binning factor", "User_Par_Name"="BINFACTOR", "User_Par_Type"="CHANNEL", "ModNum"=w468, "ChanNum"=w469) -> ()  [unwired: 9 in, 2 out]
            }
            frame #8 {
              n291 = dll-call lib="D:/Users/wymanm/Desktop/DAQuiri - 2017a/lois/Drivers/Pixie4DLL.dll" fn="_Pixie_Write_User_Par@24"("User_Par_Value"="Gate Window [µs]", "User_Par_Name"="GATE_WINDOW", "User_Par_Type"="CHANNEL", "ModNum"=w476, "ChanNum"=w475) -> ()  [unwired: 9 in, 2 out]
              n292 = dll-call lib="D:/Users/wymanm/Desktop/DAQuiri - 2017a/lois/Drivers/Pixie4DLL.dll" fn="_Pixie_Write_User_Par@24"("User_Par_Value"="Gate Delay [µs]", "User_Par_Name"="GATE_DELAY", "User_Par_Type"="CHANNEL", "ModNum"=w476, "ChanNum"=w475) -> ()  [unwired: 9 in, 2 out]
            }
            frame #9 {
              n293 = dll-call lib="D:/Users/wymanm/Desktop/DAQuiri - 2017a/lois/Drivers/Pixie4DLL.dll" fn="_Pixie_Write_User_Par@24"("User_Par_Value"="Baseline Cut", "User_Par_Name"="BLCUT", "User_Par_Type"="CHANNEL", "ModNum"=w484, "ChanNum"=w485) -> ()  [unwired: 9 in, 2 out]
              n294 = dll-call lib="D:/Users/wymanm/Desktop/DAQuiri - 2017a/lois/Drivers/Pixie4DLL.dll" fn="_Pixie_Write_User_Par@24"("User_Par_Value"="Baseline Averaging", "User_Par_Name"="BLAVG", "User_Par_Type"="CHANNEL", "ModNum"=w484, "ChanNum"=w485) -> ()  [unwired: 9 in, 2 out]
            }
            frame #10 {
              # "Update filter parameters - Module"
              n295 = dll-call lib="D:/Users/wymanm/Desktop/DAQuiri - 2017a/lois/Drivers/Pixie4DLL.dll" fn="_Pixie_Write_User_Par@24"("User_Par_Value"="Range", "User_Par_Name"="FILTER_RANGE", "User_Par_Type"="MODULE", "ModNum"=w492, "ChanNum"=0) -> ()  [unwired: 9 in, 2 out]
            }
            frame #11 {
              n296 = Boolean To (0,1)(Boolean="0 0 0 0") -> (0, 1=w566:i16)
              n297 = Boolean To (0,1)(Boolean="0 0 0 1") -> (0, 1=w565:i16)
              n298 = Boolean To (0,1)(Boolean="0 0 1 0") -> (0, 1=w564:i16)
              n299 = Boolean To (0,1)(Boolean="0 0 1 1") -> (0, 1=w563:i16)
              n300 = Boolean To (0,1)(Boolean="0 1 0 0") -> (0, 1=w562:i16)
              n301 = Boolean To (0,1)(Boolean="0 1 0 1") -> (0, 1=w561:i16)
              n302 = Boolean To (0,1)(Boolean="0 1 1 0") -> (0, 1=w560:i16)
              n303 = Boolean To (0,1)(Boolean="0 1 1 1") -> (0, 1=w559:i16)
              n304 = Multiply(x=w566, y=1) -> (x*y=w558:i32)
              n305 = Multiply(x=w565, y=2) -> (x*y=w557:i32)
              n306 = Multiply(x=w564, y=4) -> (x*y=w556:i32)
              n307 = Multiply(x=w563, y=8) -> (x*y=w555:i32)
              n308 = Multiply(x=w562, y=16) -> (x*y=w554:i32)
              n309 = Multiply(x=w561, y=32) -> (x*y=w553:i32)
              n310 = Multiply(x=w560, y=64) -> (x*y=w552:i32)
              n311 = Multiply(x=w559, y=128) -> (x*y=w551:i32)
              n312 = Add(x=w558, y=w557) -> (x+y=w504:i32)
              n313 = Add(x=w556, y=w555) -> (x+y=w550:i32)
              n314 = Add(x=w554, y=w553) -> (x+y=w549:i32)
              n315 = Add(x=w552, y=w551) -> (x+y=w505:i32)
              n316 = Add(x=w550, y=w549) -> (x+y=w506:i32)
              n317 = Add(x=w506, y=w505) -> (x+y=w503:i32)
              n318 = Add(x=w504, y=w503) -> (x+y=w497:i32)
              n319 = Boolean To (0,1)(Boolean="1 0 0 0") -> (0, 1=w532:i16)
              n320 = Boolean To (0,1)(Boolean="1 0 0 1") -> (0, 1=w531:i16)
              n321 = Boolean To (0,1)(Boolean="1 0 1 0") -> (0, 1=w530:i16)
              n322 = Boolean To (0,1)(Boolean="1 0 1 1") -> (0, 1=w529:i16)
              n323 = Boolean To (0,1)(Boolean="1 1 0 0") -> (0, 1=w528:i16)
              n324 = Boolean To (0,1)(Boolean="1 1 0 1") -> (0, 1=w527:i16)
              n325 = Boolean To (0,1)(Boolean="1 1 1 0") -> (0, 1=w526:i16)
              n326 = Boolean To (0,1)(Boolean="1 1 1 1") -> (0, 1=w525:i16)
              n327 = Multiply(x=w532, y=256) -> (x*y=w524:i32)
              n328 = Multiply(x=w531, y=512) -> (x*y=w523:i32)
              n329 = Multiply(x=w530, y=1024) -> (x*y=w522:i32)
              n330 = Multiply(x=w529, y=2048) -> (x*y=w521:i32)
              n331 = Multiply(x=w528, y=4096) -> (x*y=w520:i32)
              n332 = Multiply(x=w527, y=8192) -> (x*y=w519:i32)
              n333 = Multiply(x=w526, y=16384) -> (x*y=w518:i32)
              n334 = Multiply(x=w525, y=32768) -> (x*y=w517:i32)
              n335 = Add(x=w524, y=w523) -> (x+y=w499:i32)
              n336 = Add(x=w522, y=w521) -> (x+y=w516:i32)
              n337 = Add(x=w520, y=w519) -> (x+y=w515:i32)
              n338 = Add(x=w518, y=w517) -> (x+y=w501:i32)
              n339 = Add(x=w516, y=w515) -> (x+y=w502:i32)
              n340 = Add(x=w502, y=w501) -> (x+y=w500:i32)
              n341 = Add(x=w499, y=w500) -> (x+y=w498:i32)
              n342 = Add(x=w497, y=w498) -> (x+y=w496:i32)
              n343 = To Double Precision Float(number=w496) -> (double precision float=w495:dbl)
              n344 = dll-call lib="D:/Users/wymanm/Desktop/DAQuiri - 2017a/lois/Drivers/Pixie4DLL.dll" fn="_Pixie_Write_User_Par@24"("User_Par_Value"=w495, "User_Par_Name"="COINCIDENCE_PATTERN", "User_Par_Type"="MODULE", "ModNum"=w575, "ChanNum"=0) -> ()  [unwired: 9 in, 2 out]
            }
            frame #12 {
              n345 = Boolean To (0,1)(Boolean="Front panel contributes to STATUS line (wire-OR)") -> (0, 1=w622:i16)
              n346 = Boolean To (0,1)(Boolean="Send local hit pattern to PDM in slot 2") -> (0, 1=w618:i16)
              n347 = Boolean To (0,1)(Boolean="Front panel drives GFLT line (one module only)") -> (0, 1=w627:i16)
              n348 = Boolean To (0,1)(Boolean="Module's local test adds to global test (local fail causes global fail)") -> (0, 1=w605:i16)
              n349 = Boolean To (0,1)(Boolean="Module writes control pattern to PDM to immediate left") -> (0, 1=w620:i16)
              n350 = Multiply(x=w622, y=16384) -> (x*y=w616:i32)
              n351 = Multiply(x=w618, y=8192) -> (x*y=w613:i32)
              n352 = Multiply(x=w627, y=32) -> (x*y=w615:i32)
              n353 = Multiply(x=w605, y=4096) -> (x*y=w604:i32)
              n354 = Multiply(x=w620, y=512) -> (x*y=w614:i32)
              n355 = dll-call lib="D:/Users/wymanm/Desktop/DAQuiri - 2017a/lois/Drivers/Pixie4DLL.dll" fn="_Pixie_Read_User_Par@20"("User_Par_Name"="MODULE_CSRA", "User_Par_Type"="MODULE", "ModNum"=w579, "ChanNum"=0) -> ("User_Par_Value"=w628:dbl)  [unwired: 9 in, 2 out]
              n356 = Add(x=w615, y=w616) -> (x+y=w601:i32)
              n357 = Add(x=w604, y=w601) -> (x+y=w600:i32)
              n358 = Add(x=w614, y=w613) -> (x+y=w612:i32)
              n359 = To Unsigned Word Integer(number=w628) -> (unsigned 16bit integer=w625:u16)
              n360 = Add(x=w600, y=w612) -> (x+y=w611:i32)
              n361 = And(x=w625, y=40415) -> (x .and. y?=w610:i32)
              n362 = Add(x=w611, y=w610) -> (x+y=w609:i32)
              n363 = To Double Precision Float(number=w609) -> (double precision float=w623:dbl)
              n364 = dll-call lib="D:/Users/wymanm/Desktop/DAQuiri - 2017a/lois/Drivers/Pixie4DLL.dll" fn="_Pixie_Write_User_Par@24"("User_Par_Value"=w623, "User_Par_Name"="MODULE_CSRA", "User_Par_Type"="MODULE", "ModNum"=w579, "ChanNum"=0) -> ()  [unwired: 9 in, 2 out]
              n365 = Boolean To (0,1)(Boolean="Accept event if local pattern passes local test") -> (0, 1=w599:i16)
              n366 = Boolean To (0,1)(Boolean="Accept event if global hit pattern passes global test (in PDM)") -> (0, 1=w596:i16)
              n367 = Multiply(x=w599, y=32) -> (x*y=w598:i32)
              n368 = Multiply(x=w596, y=128) -> (x*y=w585:i32)
              n369 = dll-call lib="D:/Users/wymanm/Desktop/DAQuiri - 2017a/lois/Drivers/Pixie4DLL.dll" fn="_Pixie_Read_User_Par@20"("User_Par_Name"="MODULEPATTERN", "User_Par_Type"="MODULE", "ModNum"=w579, "ChanNum"=0) -> ("User_Par_Value"=w589:dbl)  [unwired: 9 in, 2 out]
              n370 = Add(x=w598, y=w585) -> (x+y=w581:i32)
              n371 = To Unsigned Word Integer(number=w589) -> (unsigned 16bit integer=w588:u16)
              n372 = And(x=w588, y=65375) -> (x .and. y?=w586:i32)
              n373 = Add(x=w581, y=w586) -> ()  [unwired: 1 out]
              n374 = To Double Precision Float(number=w581) -> (double precision float=w580:dbl)
              n375 = dll-call lib="D:/Users/wymanm/Desktop/DAQuiri - 2017a/lois/Drivers/Pixie4DLL.dll" fn="_Pixie_Write_User_Par@24"("User_Par_Value"=w580, "User_Par_Name"="MODULEPATTERN", "User_Par_Type"="MODULE", "ModNum"=w579, "ChanNum"=0) -> ()  [unwired: 9 in, 2 out]
            }
            frame #13 {
              n376 = Equal To 0?(x="Trigger share mode") -> (x = 0?=w660:bool)
              n377 = Equal?(x="Trigger share mode", y=1) -> (x = y?=w659:bool)
              n378 = Equal?(x="Trigger share mode", y=2) -> (x = y?=w658:bool)
              n379 = Equal?(x="Trigger share mode", y=3) -> (x = y?=w657:bool)
              n380 = case shown="True" w660 {
                tunnel: [0 0] -> w656
                frame False {
                }
                frame True {
                }
              }
              n381 = case shown="True" w659 {
                tunnel: [0 4] -> w655
                frame False {
                }
                frame True {
                }
              }
              n382 = case shown="True" w658 {
                tunnel: [0 32768] -> w654
                frame False {
                }
                frame True {
                }
              }
              n383 = case shown="True" w657 {
                tunnel: [0 32772] -> w653
                frame False {
                }
                frame True {
                }
              }
              n384 = Add(x=w656, y=w655) -> (x+y=w652:i32)
              n385 = Add(x=w654, y=w653) -> (x+y=w651:i32)
              n386 = Add(x=w652, y=w651) -> (x+y=w642:i32)
              n387 = To Double Precision Float(number="PDM control pattern") -> (double precision float=w664:dbl)
              n388 = dll-call lib="D:/Users/wymanm/Desktop/DAQuiri - 2017a/lois/Drivers/Pixie4DLL.dll" fn="_Pixie_Read_User_Par@20"("User_Par_Name"="MODULE_CSRA", "User_Par_Type"="MODULE", "ModNum"=w638, "ChanNum"=0) -> ("User_Par_Value"=w646:dbl)  [unwired: 9 in, 2 out]
              n389 = To Unsigned Word Integer(number=w646) -> (unsigned 16bit integer=w645:u16)
              n390 = dll-call lib="D:/Users/wymanm/Desktop/DAQuiri - 2017a/lois/Drivers/Pixie4DLL.dll" fn="_Pixie_Write_User_Par@24"("User_Par_Value"=w664, "User_Par_Name"="NNSHAREPATTERN", "User_Par_Type"="MODULE", "ModNum"=w638, "ChanNum"=0) -> ()  [unwired: 9 in, 2 out]
              n391 = And(x=w645, y=32763) -> (x .and. y?=w643:i32)
              n392 = Add(x=w642, y=w643) -> (x+y=w637:i32)
              n393 = To Double Precision Float(number=w637) -> (double precision float=w636:dbl)
              n394 = dll-call lib="D:/Users/wymanm/Desktop/DAQuiri - 2017a/lois/Drivers/Pixie4DLL.dll" fn="_Pixie_Write_User_Par@24"("User_Par_Value"=w636, "User_Par_Name"="MODULE_CSRA", "User_Par_Type"="MODULE", "ModNum"=w638, "ChanNum"=0) -> ()  [unwired: 9 in, 2 out]
            }
            frame #14 {
              # "ALWAYS CLEAR BIT 0 of DblbufCSR"
              n395 = Boolean To (0,1)(Boolean="32 buffers per spill") -> (0, 1=w698:i16)
              n396 = Multiply(x=w698, y=2) -> (x*y=w694:i32)
              n397 = dll-call lib="D:/Users/wymanm/Desktop/DAQuiri - 2017a/lois/Drivers/Pixie4DLL.dll" fn="_Pixie_Read_User_Par@20"("User_Par_Name"="MODULE_CSRA", "User_Par_Type"="MODULE", "ModNum"=w677, "ChanNum"=0) -> ("User_Par_Value"=w701:dbl)  [unwired: 9 in, 2 out]
              n398 = To Unsigned Word Integer(number=w701) -> (unsigned 16bit integer=w700:u16)
              n399 = And(x=w700, y=65533) -> (x .and. y?=w695:i32)
              n400 = Add(x=w694, y=w695) -> (x+y=w693:i32)
              n401 = To Double Precision Float(number=w693) -> (double precision float=w689:dbl)
              n402 = dll-call lib="D:/Users/wymanm/Desktop/DAQuiri - 2017a/lois/Drivers/Pixie4DLL.dll" fn="_Pixie_Write_User_Par@24"("User_Par_Value"=w689, "User_Par_Name"="MODULE_CSRA", "User_Par_Type"="MODULE", "ModNum"=w677, "ChanNum"=0) -> ()  [unwired: 9 in, 2 out]
              n403 = dll-call lib="D:/Users/wymanm/Desktop/DAQuiri - 2017a/lois/Drivers/Pixie4DLL.dll" fn="_Pixie_Read_User_Par@20"("User_Par_Name"="DBLBUFCSR", "User_Par_Type"="MODULE", "ModNum"=w677, "ChanNum"=0) -> ("User_Par_Value"=w685:dbl)  [unwired: 9 in, 2 out]
              n404 = To Unsigned Word Integer(number=w685) -> (unsigned 16bit integer=w684:u16)
              n405 = And(x=w684, y=65534) -> (x .and. y?=w679:i32)
              n406 = To Double Precision Float(number=w679) -> (double precision float=w678:dbl)
              n407 = dll-call lib="D:/Users/wymanm/Desktop/DAQuiri - 2017a/lois/Drivers/Pixie4DLL.dll" fn="_Pixie_Write_User_Par@24"("User_Par_Value"=w678, "User_Par_Name"="DBLBUFCSR", "User_Par_Type"="MODULE", "ModNum"=w677, "ChanNum"=0) -> ()  [unwired: 9 in, 2 out]
            }
          }
        }
        frame False {
        }
      }
    }
  }
